vi "Send command Get Pin.vi"(7 "Marca":string, 8 "error in (no error)":errorcluster, 9 "Pin":string, 10 "Puerto":string, 11 "Arduino in":refnum<class "Arduino.lvclass">) -> (0 "error out":errorcluster, 1 "Command":string, 2 "Expected response":string, 3 "Arduino out":refnum<class "Arduino.lvclass">)   [LabVIEW 2020, in "Arduino.lvclass"]
uses:
  Arduino.lvclass
  D:/Fork/IVProyecto_3P/Abstract/Serial Device/Serial Device.lvclass
  Arduino.lvclass/Arduino.ctl
  Abstract/Serial Device/Serial Device.lvclass
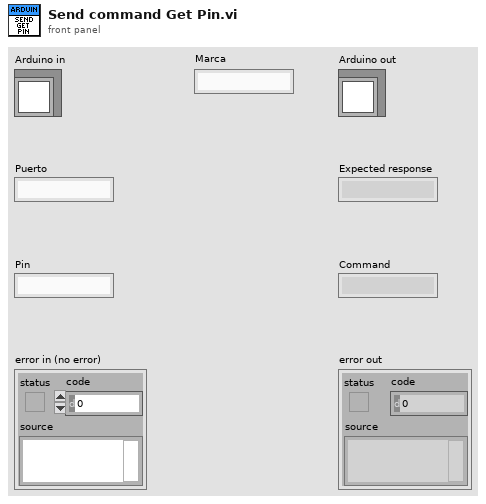
[diagram p1: front panel]
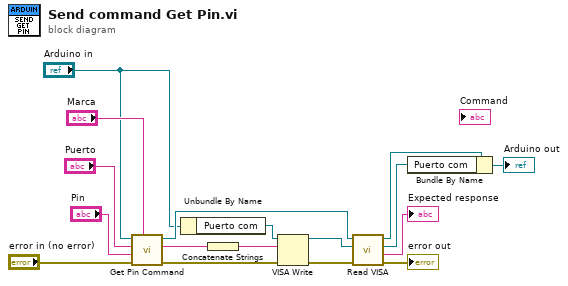
[diagram p0: block diagram]
diagram:
  n1 = call "Get Pin Command.vi"("Marca"="Marca", "error in (no error)"="error in (no error)", "Pin"="Pin", "Puerto"="Puerto", "Serial Device in"="Arduino in") -> ("error out"=w9:errorcluster, "Command"=w10:string, "Serial Device out"=w11:refnum<class "Arduino.lvclass">)  [unwired: 3 in, 1 out]
  n2 = Unbundle By Name("Arduino in") -> ("Puerto com"=w15:refnum<visa-resource-name>)
  n3 = Concatenate Strings(w10) -> (w16:string)
  n4 = VISA Write(VISA resource name=w15, write buffer=w16, error in (no error)=w9) -> (VISA resource name out=w14:refnum<visa-resource-name>, error out=w17:errorcluster)  [unwired: 1 out]
  n5 = call-dynamic "Read VISA.vi"("error in (no error)"=w17, "VISA Refnum in"=w14, "Serial Device in"=w11) -> ("error out"=→"error out":errorcluster, "Serial Response"=→"Expected response":string, "VISA resource name out"=w12:refnum<visa-resource-name>, "Serial Device out"=w13:refnum<class "Arduino.lvclass">)  [unwired: 5 in]
  n6 = Bundle By Name(cluster=w13, "Puerto com"=w12) -> (→"Arduino out":refnum<class "Arduino.lvclass">)
